vi "Initialize.vi"(8 "error in (no error)":errorcluster, 11 "G-UE in":refnum<class "G-UE.lvclass">) -> (0 "error out":errorcluster, 3 "G-UE out":refnum<class "G-UE.lvclass">)   [LabVIEW 2016, in "G-UE.lvclass"]
uses:
  G-UE.lvclass
  <vilib>/Analysis/Matrix/Datatypes/ComplexMatrix.ctl
  G-UE.lvclass/G-UE.ctl
  <vilib>/Analysis/Matrix/NI_Matrix.lvlib
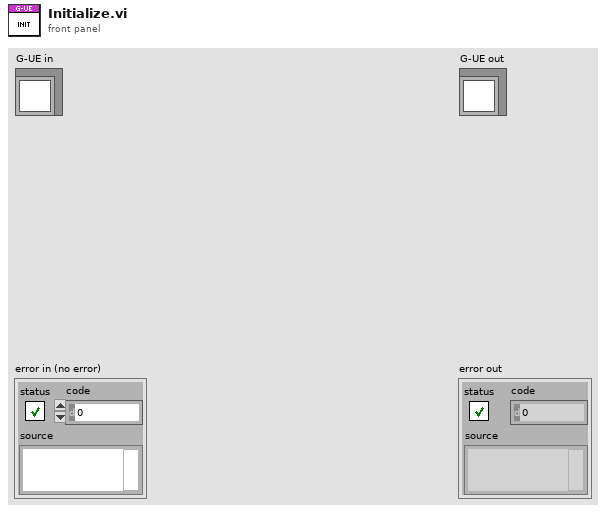
[diagram p1: front panel]
types:
  T1 = typedef "NI_Matrix.lvlib/ComplexMatrix.ctl" = cdb[][]
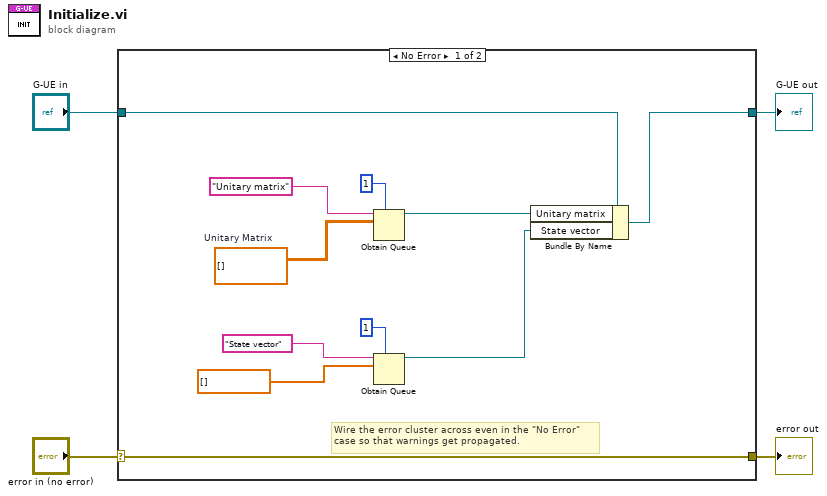
[diagram p0: block diagram]
diagram:
  n1 = case shown="No Error" "error in (no error)" {
    selector: "error in (no error)" -> [w15 w17]
    tunnel: [w15 w17] -> w3
    tunnel: [w13 w16] -> w1
    tunnel: "G-UE in" -> [w14 w16]
    frame No Error {
      w9 = T1 []  # Unitary Matrix
      # "Wire the error cluster across even in the \"No Error\"\ncase so that warnings get propagated."
      n2 = Obtain Queue(max queue size (-1, unlimited)=1, name (unnamed)="Unitary matrix", element data type=w9) -> (queue out=w6:refnum<queue>)  [unwired: 2 in, 2 out]
      n3 = Obtain Queue(max queue size (-1, unlimited)=1, name (unnamed)="State vector", element data type=cdb[] [] ("subarray")) -> (queue out=w5:refnum<queue>)  [unwired: 2 in, 2 out]
      n4 = Bundle By Name(cluster=w14, "Unitary matrix"=w6, "State vector"=w5) -> (w13:refnum<class "G-UE.lvclass">)
    }
    frame Error {
    }
  }
  "error out" <- w3
  "G-UE out" <- w1
